vi "4Pi Capture Write Meta Data.vi"(11 "data path":path) -> ()   [LabVIEW 2021]
uses:
  <vilib>/regexp/Match Regular Expression.xnode
  <vilib>/Utility/config.llb/NI_LVConfig.lvlib
  <vilib>/Utility/Data Type/NI_Data Type.lvlib
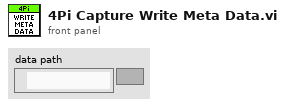
[diagram p1: front panel]
types:
  T1 = enum16{"open", "replace", "create", "open or create", "replace or create", "replace or create with confirmation"}
  T2 = typedef "NI_LVConfig.lvlib/Config Data RefNum.ctl" = refnum<k1>
  T3 = cluster{"VI Path":path, "VI Refnum":refnum<vi>}[]
  T4 = typedef "NI_Data Type.lvlib/Data Type.ctl" = enum8{"Invalid Type", "Void", "I8", "I16", "I32", "I64", "U8", "U16", "U32", "U64", "Single Float", "Double Float", "Extended Float", "Single Complex", "Double Complex", "Extended Complex", "Enum U8", "Enum U16", "Enum U32", "Enum U64", "Single Float With Unit", "Double Float With Unit", "Extended Float With Unit", "Single Complex with Unit", "Double Complex with Unit", "Extended Complex with Unit", "Boolean", "String", "Path", "Picture", "Tag", "Array", "Cluster", "Variant", "LV Variant", "Waveform", "Timestamp", "Digital Waveform", "Digital Data", "ExpressData", "Refnum", "External Data", "VI", "Poly VI", "LabVIEW Class Instance", "Fixed Point", "Set Collection", "Map Collection"}
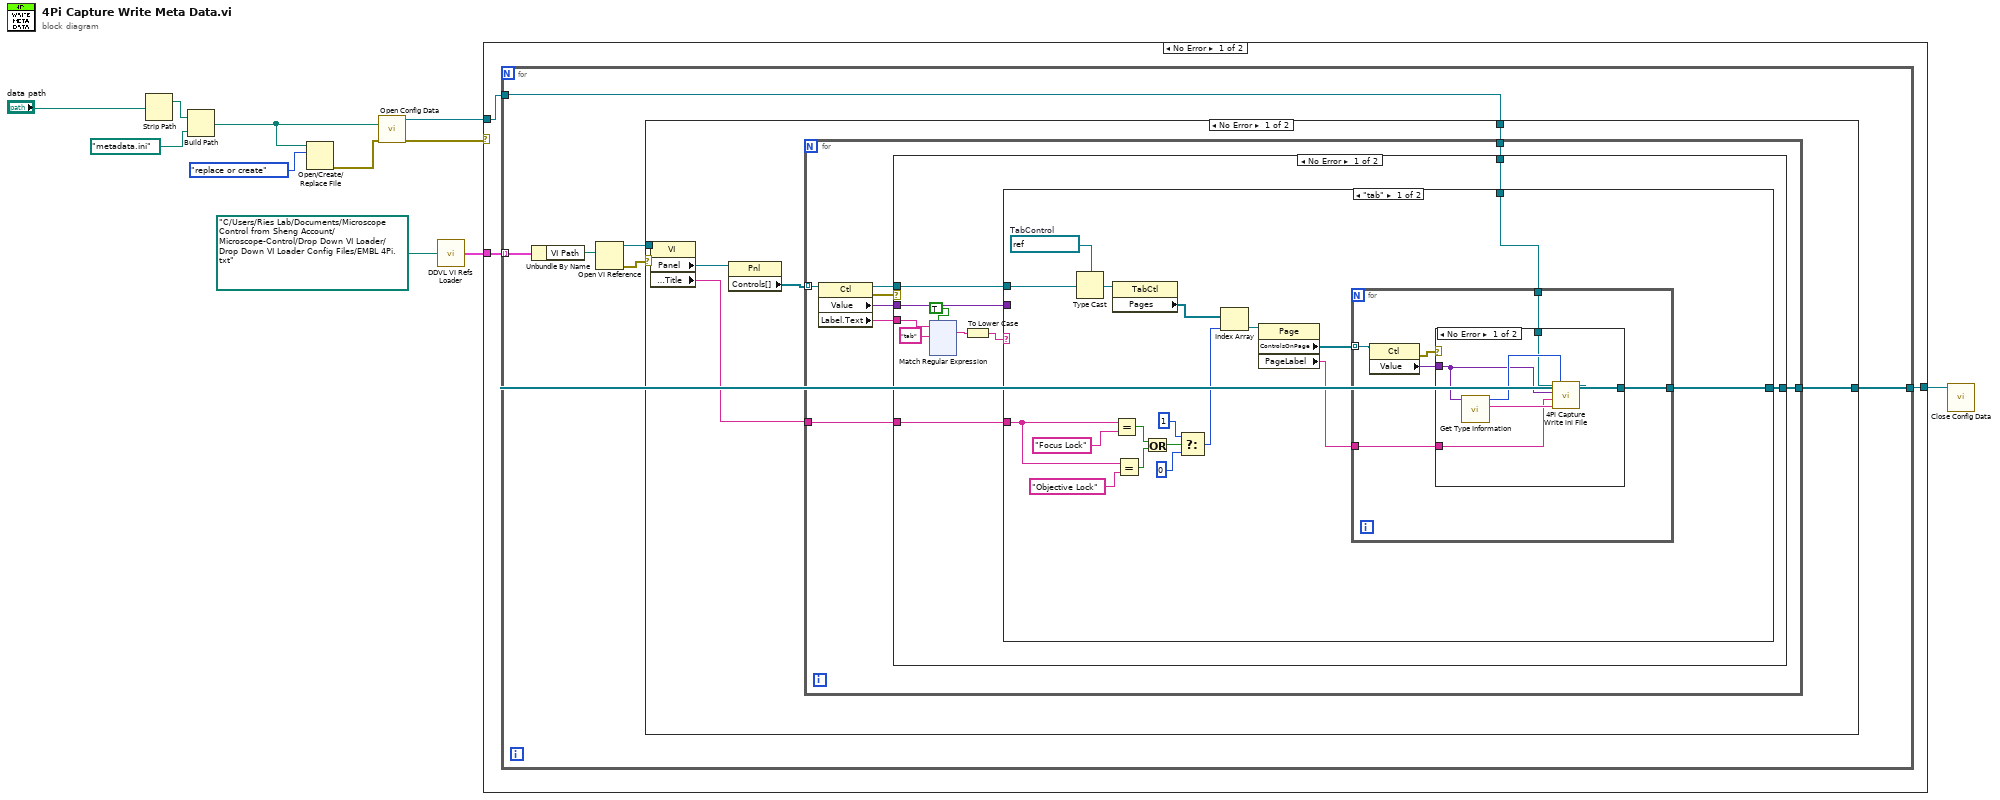
[diagram p0: block diagram]
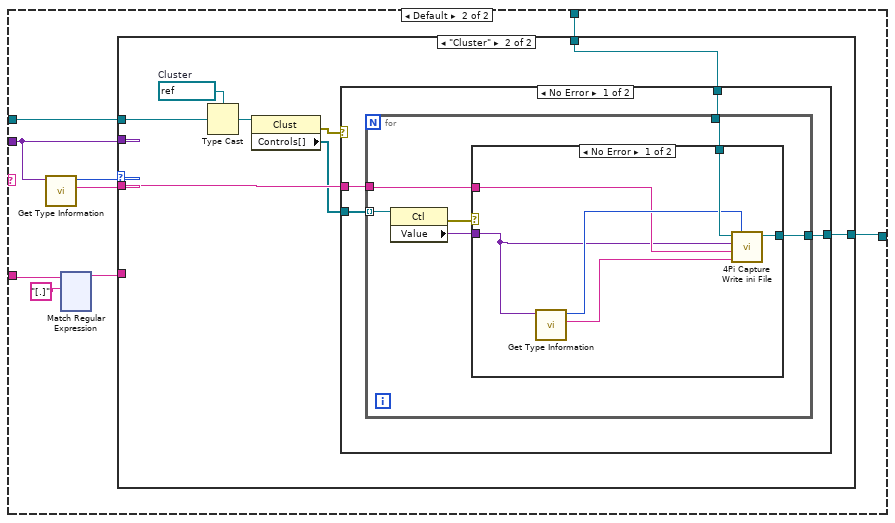
[diagram p3: hidden frame]
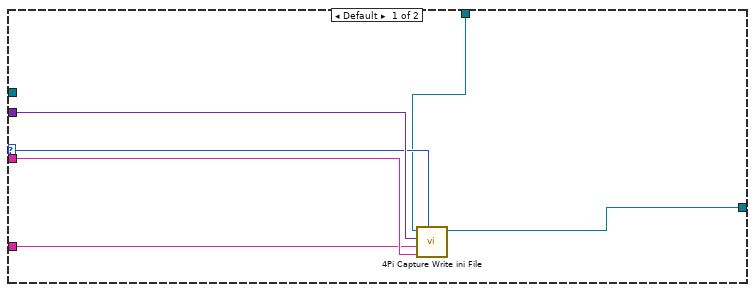
[diagram p4: hidden frame]
diagram:
  n1 = Strip Path(path="data path") -> (stripped path=w10:path)  [unwired: 1 out]
  n2 = Build Path(base path=w10, name or relative path=path "metadata.ini" ("default name")) -> (appended path=w4:path)
  n3 = Open/Create/Replace File(file path (use dialog)=w4, operation (0:open)=T1."replace or create") -> (error out=w5:errorcluster)  [unwired: 4 in, 2 out]
  n4 = call <vilib>:"Open Config Data.vi"("error in (no error)"=w5, "configuration file path"=w4) -> ("error out"=w2:errorcluster, "refnum"=w1:T2)  [unwired: 1 in, 7 out]
  n5 = call "DDVL VI Refs Loader.vi"("Config File Path"=path "C:/Users/Ries Lab/Documents/Microscope Control from Sheng Account/Microscope-Control/Drop Down VI Loader/Drop Down VI Loader Config Files/EMBL 4Pi.txt") -> ("VI Path/Ref"=w8:T3)  [unwired: 12 in, 2 out]
  n6 = case shown="No Error" w2 {
    tunnel: [w14 w353] -> w9
    tunnel: w8 -> [w13 _]
    tunnel: w1 -> [w12 w353]
    frame No Error {
      n7 = for {
        tunnel: [w19] -> w14
        tunnel: w13 -> [w18] mode=indexing
        tunnel: w12 -> [w15]
        n8 = Unbundle By Name(w18) -> ("VI Path"=w17:path)
        n9 = Open VI Reference(vi path=w17) -> (vi reference=w20:refnum<vi>, error out=w16:errorcluster)  [unwired: 5 in]
        n10 = case shown="No Error" w16 {
          tunnel: w20 -> [w26 _]
          tunnel: [w23 w352] -> w19
          tunnel: w15 -> [w21 w352]
          frame No Error {
            n11 = property class="VI"(reference=w26) -> ("Panel"=w25:refnum<vi>, "Front Panel.Title"=w22:string)  [unwired: 1 in, 2 out]
            n12 = property class="Pnl"(reference=w25) -> ("Controls[]"=w24:refnum<vi>[])  [unwired: 1 in, 2 out]
            n13 = for {
              tunnel: w24 -> [w34] mode=indexing
              tunnel: [w32] -> w23
              tunnel: w22 -> [w31]
              tunnel: w21 -> [w27]
              n14 = property class="Ctl"(reference=w34) -> (reference out=w29:refnum<vi>, error out=w28:errorcluster, "Value"=w33:variant, "Label.Text"=w30:string)  [unwired: 1 in]
              n15 = case shown="No Error" w28 {
                tunnel: w33 -> [w44 _]
                tunnel: [w43 w351] -> w32
                tunnel: w31 -> [w42 _]
                tunnel: w30 -> [w41 _]
                tunnel: w29 -> [w38 _]
                tunnel: w27 -> [w35 w351]
                frame No Error {
                  n16 = xnode "Match Regular Expression"("input string"=w41, "regular expression"="tab", "ignore case? (F)"=TRUE) -> ("whole match"=w37:string)  [unwired: 3 in, 4 out]
                  n17 = To Lower Case(string=w37) -> (all lower case string=w36:string)
                  n18 = case shown="\"tab\"" w36 {
                    tunnel: w44 -> [_ w198]
                    tunnel: [w172 w194] -> w43
                    tunnel: w42 -> [w164 w200]
                    tunnel: w38 -> [w175 w199]
                    tunnel: w35 -> [w162 w193]
                    frame "tab" {
                      w179 = refnum<vi> refnum  # TabControl
                      n19 = Type Cast(type=w179, x=w175) -> (*(type *) &x=w178:refnum<vi>)
                      n20 = property class="TabCtl"(reference=w178) -> ("Pages"=w176:refnum<vi>[])  [unwired: 1 in, 2 out]
                      n21 = Equal?(x=w164, y="Focus Lock") -> (x = y?=w168:bool)
                      n22 = Equal?(x=w164, y="Objective Lock") -> (x = y?=w167:bool)
                      n23 = Or(x=w168, y=w167) -> (x .or. y?=w169:bool)
                      n24 = Select(t=1 ("index"), s=w169, f=0) -> (s? t:f=w163:i32)
                      n25 = Index Array(array=w176, index=w163) -> (element=w177:refnum<vi>)
                      n26 = property class="Page"(reference=w177) -> ("ControlsOnPage"=w174:refnum<vi>[], "PageLabel"=w173:string)  [unwired: 1 in, 2 out]
                      n27 = for {
                        tunnel: w174 -> [w185] mode=indexing
                        tunnel: w173 -> [w180]
                        tunnel: w162 -> [w184]
                        tunnel: [w182] -> w172
                        n28 = property class="Ctl"(reference=w185) -> (error out=w181:errorcluster, "Value"=w183:variant)  [unwired: 1 in, 1 out]
                        n29 = case shown="No Error" w181 {
                          tunnel: w184 -> [w190 w192]
                          tunnel: w180 -> [w188 _]
                          tunnel: w183 -> [w187 _]
                          tunnel: [w186 w192] -> w182
                          frame No Error {
                            n30 = call <vilib>:"Get Type Information.vi"("variant"=w187) -> ("name"=w189:string, "type"=w191:T4)  [unwired: 6 in, 3 out]
                            n31 = call "4Pi Capture Write ini File.vi"("type"=w191, "property name"=w189, "section name"=w188, "Variant"=w187, "Refnum in"=w190) -> ("Refnum out"=w186:T2)  [unwired: 5 in, 1 out]
                          }
                          frame Error {
                          }
                        }
                      }
                    }
                    frame Default {
                      n32 = call <vilib>:"Get Type Information.vi"("variant"=w198) -> ("name"=w196:string, "type"=w197:T4)  [unwired: 6 in, 3 out]
                      n33 = xnode "Match Regular Expression"("input string"=w200, "regular expression"="[.]") -> ("before match"=w195:string)  [unwired: 4 in, 4 out]
                      n34 = case shown="\"Cluster\"" w197 {
                        selector: w197 -> [w205 _]
                        tunnel: w198 -> [w207 _]
                        tunnel: w196 -> [w204 w214]
                        tunnel: [w206 w215] -> w194
                        tunnel: w195 -> [w203 _]
                        tunnel: w199 -> [_ w211]
                        tunnel: w193 -> [w202 w208]
                        frame Default {
                          n35 = call "4Pi Capture Write ini File.vi"("type"=w205, "property name"=w204, "section name"=w203, "Variant"=w207, "Refnum in"=w202) -> ("Refnum out"=w206:T2)  [unwired: 5 in, 1 out]
                        }
                        frame "Cluster" {
                          w212 = refnum<vi> refnum  # Cluster
                          n36 = Type Cast(type=w212, x=w211) -> (*(type *) &x=w213:refnum<vi>)
                          n37 = property class="Clust"(reference=w213) -> (error out=w209:errorcluster, "Controls[]"=w210:refnum<vi>[])  [unwired: 1 in, 1 out]
                          n38 = case shown="No Error" w209 {
                            tunnel: w208 -> [w219 w233]
                            tunnel: [w218 w233] -> w215
                            tunnel: w214 -> [w217 _]
                            tunnel: w210 -> [w216 _]
                            frame No Error {
                              n39 = for {
                                tunnel: w219 -> [w225]
                                tunnel: [w224] -> w218
                                tunnel: w217 -> [w223]
                                tunnel: w216 -> [w222] mode=indexing
                                n40 = property class="Ctl"(reference=w222) -> (error out=w220:errorcluster, "Value"=w221:variant)  [unwired: 1 in, 1 out]
                                n41 = case shown="No Error" w220 {
                                tunnel: w225 -> [w231 w232]
                                tunnel: [w230 w232] -> w224
                                tunnel: w223 -> [w227 _]
                                tunnel: w221 -> [w226 _]
                                frame No Error {
                                n42 = call <vilib>:"Get Type Information.vi"("variant"=w226) -> ("name"=w228:string, "type"=w229:T4)  [unwired: 6 in, 3 out]
                                n43 = call "4Pi Capture Write ini File.vi"("type"=w229, "property name"=w228, "section name"=w227, "Variant"=w226, "Refnum in"=w231) -> ("Refnum out"=w230:T2)  [unwired: 5 in, 1 out]
                                }
                                frame Error {
                                }
                                }
                              }
                            }
                            frame Error {
                            }
                          }
                        }
                      }
                    }
                  }
                }
                frame Error {
                }
              }
            }
          }
          frame Error {
          }
        }
      }
    }
    frame Error {
    }
  }
  n44 = call <vilib>:"Close Config Data.vi"("refnum"=w9) -> ()  [unwired: 2 in, 9 out]
